vi "Set Multi Track.vi"(6 "gap":i32, 7 "bottom":i32, 9 "offset":i32, 10 "height":i32, 11 "number":i32) -> (3 "function return":u32, 4 "gap out":i32, 5 "bottom out":i32)   [LabVIEW 2018, in "Copy of Andor SDK.lvlib"]
doc: "EXPNETTYPE unsigned int WINAPI SetMultiTrack(int number, int height, int offset, int * bottom, int * gap);"
uses:
  Copy of Andor SDK.lvlib
  <userlib>/Andor SDK/ATMCD32D.dll
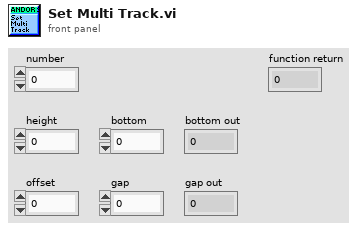
[diagram p1: front panel]
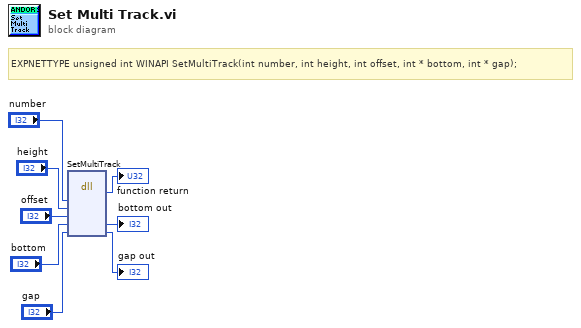
[diagram p0: block diagram]
diagram:
  # "EXPNETTYPE unsigned int WINAPI SetMultiTrack(int number, int height, int offset, int * bottom, int * gap);"
  n1 = dll-call lib="C:/Program Files (x86)/National Instruments/LabVIEW 2018/user.lib/Andor SDK/ATMCD32D.*" fn="SetMultiTrack"("number"="number", "height"="height", "offset"="offset", "bottom"="bottom", "gap"="gap") -> (→"function return":u32, "bottom"=→"bottom out":i32, "gap"=→"gap out":i32)  [unwired: 6 in, 2 out]
